vi "TX-SIS-BPCS-Modbus (SubVI).vi"(6 "SIS-10SDV502":bool, 8 "error in (no error)":errorcluster, 9 "SIS-10SDV501":bool, 10 "SIS-10SDV500":bool, 11 "Modbus Slave in":refnum<class "Modbus Slave.lvclass">) -> (0 "error out":errorcluster, 2 "TX-SIS-BPCS-ARRAY":bool[](array[boolean]), 3 "Modbus Slave out":refnum<class "Modbus Slave.lvclass">)   [LabVIEW 2018]
uses:
  <vilib>/Modbus/slave/Modbus Slave.lvclass
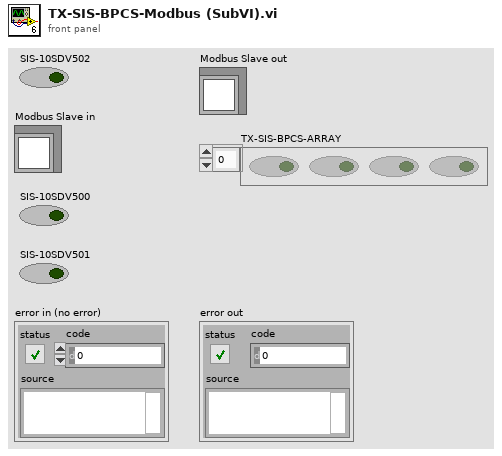
[diagram p1: front panel]
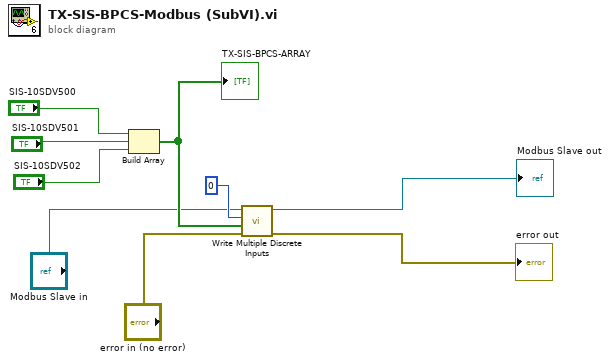
[diagram p0: block diagram]
diagram:
  n1 = Build Array("SIS-10SDV500", "SIS-10SDV501", "SIS-10SDV502") -> (w7:bool[])
  "TX-SIS-BPCS-ARRAY" <- w7
  n2 = call-dynamic "Write Multiple Discrete Inputs.vi"("error in (no error)"="error in (no error)", "discrete input values"=w7, "starting address"=u16 0, "Modbus slave in"="Modbus Slave in") -> ("error out"=→"error out":errorcluster, "Modbus slave out"=→"Modbus Slave out":refnum<class "Modbus Slave.lvclass">)  [unwired: 6 in]
